vi "Configure and read.vi"(6 "error in":errorcluster, 8 "Configuration":T1, 9 "VISA resource name":refnum<visa-resource-name>) -> (0 "error out":errorcluster, 2 "Read value":string, 3 "VISA resource name out":refnum<visa-resource-name>)   [LabVIEW 2023, in "Aim TTi 1908P DMM.lvlib"]
uses:
  Aim TTi 1908P DMM.lvlib
  34c442d0-076a-446d-8d09-49ed1551a703.vi
  Configure.ctl
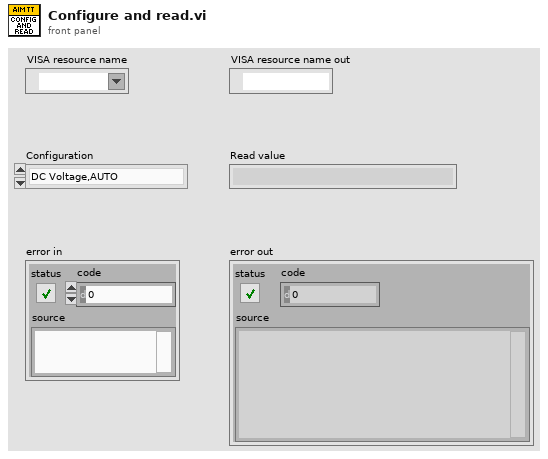
[diagram p1: front panel]
types:
  T1 = typedef "Aim TTi 1908P DMM.lvlib/Configure.ctl" = enum16{"DC Voltage,AUTO", "DC Voltage, 100V", "DC Voltage,10V", "Resistance,AUTO", "Resistance,10K"}
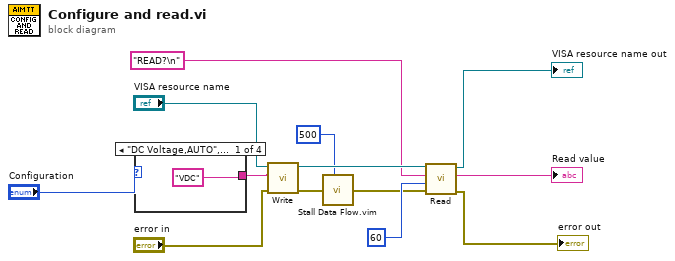
[diagram p0: block diagram]
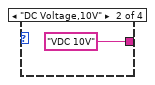
[diagram p2: hidden frame]
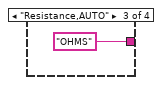
[diagram p3: hidden frame]
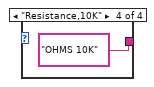
[diagram p4: hidden frame]
diagram:
  n1 = case shown="\"DC Voltage,AUTO\", Default" "Configuration" {
    tunnel: ["VDC" ("Data to write") "VDC 10V" ("Data to write") "OHMS" ("Data to write") "OHMS 10K" ("Data to write")] -> w10
    frame "DC Voltage,AUTO", Default {
    }
    frame "DC Voltage,10V" {
    }
    frame "Resistance,AUTO" {
    }
    frame "Resistance,10K" {
    }
  }
  n2 = call "Write.vi"("error in"="error in", "Data to write"=w10, "VISA resource name"="VISA resource name") -> ("error out"=w8:errorcluster, "VISA resource name out"=w12:refnum<visa-resource-name>)  [unwired: 5 in]
  n3 = call "Stall Data Flow.vim"("value in"=w8, "milliseconds to wait"=u32 500) -> ("value out"=w2:errorcluster)  [unwired: 1 out]
  n4 = call "Read.vi"("error in"=w2, "byte count"=u32 60, "Read command"="READ?\n", "VISA resource name"=w12) -> ("error out"=→"error out":errorcluster, "Read data"=→"Read value":string, "VISA resource name out"=→"VISA resource name out":refnum<visa-resource-name>)  [unwired: 3 in]
